vi "Close.vi"(8 "error in (no error)":errorcluster, 11 "ASIA Pump C":T1 {"channel" min=0 max=1 step=1}) -> (0 "error out":errorcluster, 2 "Task Completed":bool, 3 "ASIA Pump C":T1 {"channel" min=0 max=1 step=1})   [LabVIEW 2018, in "ASIA Pump.lvlib"]
uses:
  ASIA Pump.lvlib
  Pump Settings.ctl
panel:
  out "path out":path
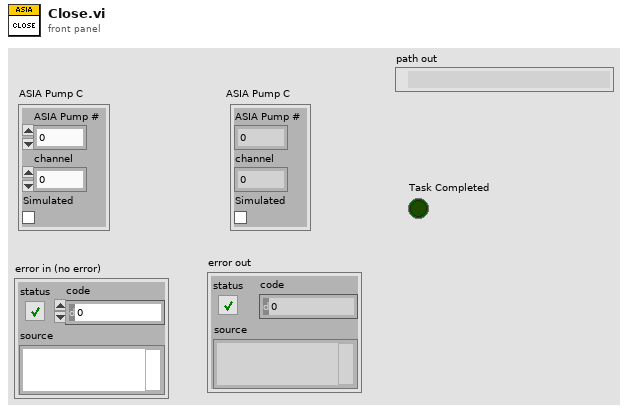
[diagram p1: front panel]
types:
  T1 = typedef "ASIA Pump.lvlib/Pump Settings.ctl" = cluster{"ASIA Pump #":i32, "channel":i32, "Simulated":bool}
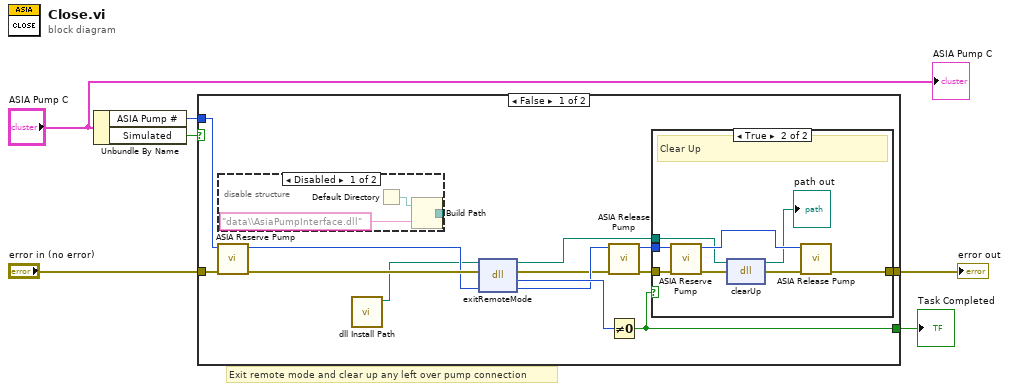
[diagram p0: block diagram]
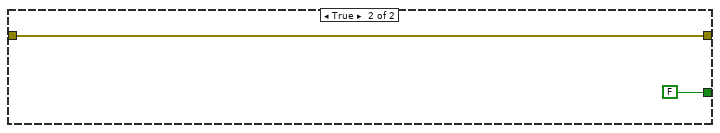
[diagram p4: hidden frame]
diagram:
  # "Exit remote mode and clear up any left over pump connection"
  n1 = Unbundle By Name("ASIA Pump C") -> ("ASIA Pump #"=w2:i32, "Simulated"=w1:bool)
  n2 = case shown="False" w1 {
    tunnel: "error in (no error)" -> [w16 w33]
    tunnel: w2 -> [w14 _]
    tunnel: [w19 w33] -> w4
    tunnel: [w17 FALSE] -> w3
    frame False {
      n3 = call "ASIA Reserve Pump.vi"("error in (no error)"=w16, "ASIA Pump # In"=w14) -> ("error out"=w15:errorcluster, "ASIA Pump # Out"=w13:i32)  [unwired: 8 in]
      n4 = disable-structure shown="Disabled" {
        disable-tunnel: [w20 _] -> _
        frame Disabled {
          n5 = Default Directory() -> (w21:path)
          n6 = Build Path(base path=w21, name or relative path="data\\AsiaPumpInterface.dll") -> (appended path=w20:path)
        }
        frame Enabled {
        }
      }
      n7 = call "dll Install Path.vi"() -> ("system directory"=w8:path)  [unwired: 11 in]
      n8 = dll-call lib="C:/Program Files (x86)/Pfizer/FAST/data/AsiaPumpInterface.dll" fn="exitRemoteMode"(path in=w8, error in=w15, "pumpNum"=w13) -> (path out=w7:path, error out=w11:errorcluster, "Bool"=w18:u8, "pumpNum"=w12:u32)  [unwired: 1 in]
      n9 = call "ASIA Release Pump.vi"("error in (no error)"=w11, "pumpNum"=w12) -> ("error out"=w10:errorcluster, "ASIA Pump # Out"=w9:i32)  [unwired: 8 in]
      n10 = Not Equal To 0?(x=w18) -> (x != 0?=w17:bool)
      n11 = case shown="True" w17 {
        tunnel: w10 -> [w23 w31]
        tunnel: [w23 w26] -> w19
        tunnel: w9 -> [_ w29]
        tunnel: w7 -> [_ w25]
        frame False {
          # "Error"
        }
        frame True {
          # "Clear Up"
          n12 = call "ASIA Reserve Pump.vi"("error in (no error)"=w31, "ASIA Pump # In"=w29) -> ("error out"=w30:errorcluster, "ASIA Pump # Out"=w28:i32)  [unwired: 8 in]
          n13 = dll-call lib="C:/Program Files (x86)/Pfizer/FAST/data/AsiaPumpInterface.dll" fn="clearUp"(path in=w25, error in=w30) -> (path out=→"path out":path, error out=w27:errorcluster)  [unwired: 2 in]
          n14 = call "ASIA Release Pump.vi"("error in (no error)"=w27, "pumpNum"=w28) -> ("error out"=w26:errorcluster)  [unwired: 8 in, 1 out]
        }
      }
    }
    frame True {
    }
  }
  "error out" <- w4
  "Task Completed" <- w3
  "ASIA Pump C" <- "ASIA Pump C"
